vi "TimeTagToTimeStamp.vi"(11 "time tag in":u32[](array[numeric]) format="%.0x") -> (2 "nSec counter":u64[](array[numeric]), 3 "time stamp":timestamp[](array[timestamp]))   [LabVIEW 2020, in "AIM664LV.lvlib"]
uses:
  AIM664LV.lvlib
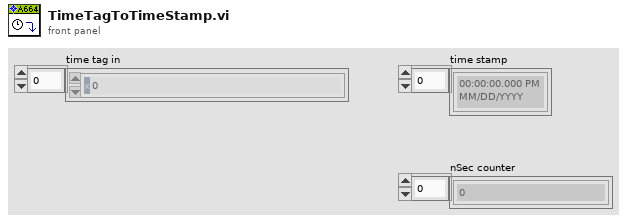
[diagram p1: front panel]
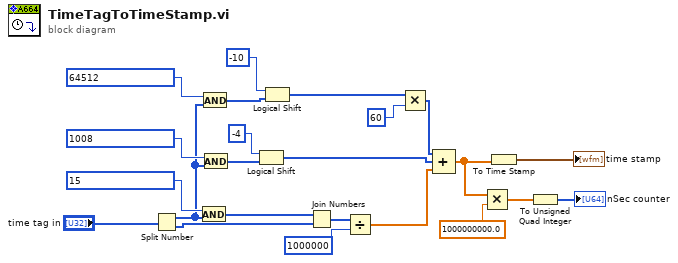
[diagram p0: block diagram]
diagram:
  n1 = Split Number(x="time tag in") -> (hi(x)=w16:u16[], lo(x)=w19:u16[])
  n2 = And(x=u16 15, y=w16) -> (x .and. y?=w20:u16[])
  n3 = And(x=u16 64512, y=w16) -> (x .and. y?=w13:u16[])
  n4 = And(x=u16 1008, y=w16) -> (x .and. y?=w15:u16[])
  n5 = Logical Shift(y=i16 -4, x=w15) -> (x << y=w7:u16[])
  n6 = Logical Shift(y=i16 -10, x=w13) -> (x << y=w11:u16[])
  n7 = Join Numbers(hi=w20, lo=w19) -> ((hi.lo)=w5:u32[])
  n8 = Divide(x=w5, y=u32 1000000) -> (x/y=w9:dbl[])
  n9 = Multiply(x=w11, y=u16 60) -> (x*y=w8:u16[])
  n10 = Compound Arithmetic op=ADD(w8, w7, w9) -> (w4:dbl[])
  n11 = Multiply(x=w4, y=1000000000.0) -> (x*y=w2:dbl[])
  n12 = To Time Stamp(1:w4) -> (0:→"time stamp":timestamp[])
  n13 = To Unsigned Quad Integer(1:w2) -> (0:→"nSec counter":u64[])
